vi "HMGET.vi"(8 "error in (no error)":errorcluster, 9 "fields":string[](array[string]), 10 "key":string, 11 "Redis Client in":refnum<class "Redis Client.lvclass">) -> (0 "error out":errorcluster, 1 "found?":bool, 2 "RESP3 Values out":variant[](array[variant]), 3 "Redis Client out":refnum<class "Redis Client.lvclass">)   [LabVIEW 2019, in "Redis Client for LabVIEW.lvlib" / "Redis Client.lvclass"]
uses:
  Redis Client.lvclass
  lib/RESP3-for-LabVIEW/RESP3/subVIs/RESP3 Make String Base.vi
  lib/RESP3-for-LabVIEW/RESP3/types/RESP3 data type attribute.vi
  lib/RESP3-for-LabVIEW/RESP3/RESP3.lvlib
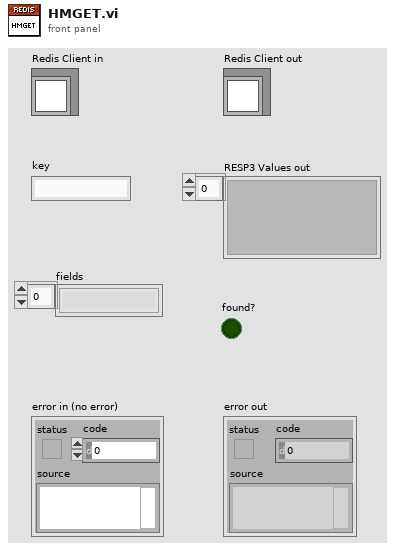
[diagram p1: front panel]
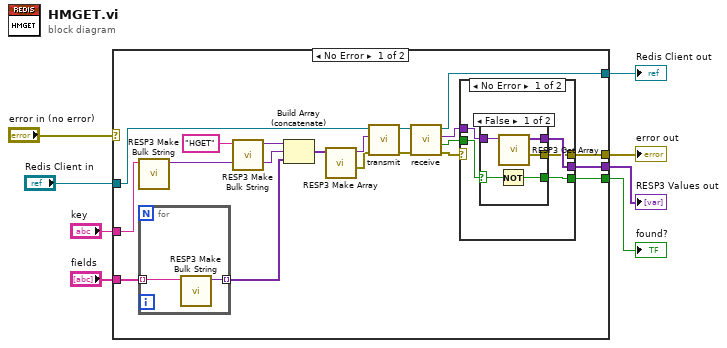
[diagram p0: block diagram]
diagram:
  n1 = case shown="No Error" "error in (no error)" {
    selector: "error in (no error)" -> [_ w42]
    tunnel: [w14 w42] -> w7
    tunnel: "Redis Client in" -> [w27 w41]
    tunnel: [w24 w41] -> w5
    tunnel: "key" -> [w21 _]
    tunnel: "fields" -> [w20 _]
    tunnel: [w13 _] -> w2
    tunnel: [w10 _] -> w1
    frame No Error {
      n2 = call "RESP3 Make Bulk String.vi"("String"=w21) -> ("RESP3 Value out"=w18:variant)  [unwired: 9 in, 1 out]
      n3 = for {
        tunnel: w20 -> [w29] mode=indexing
        tunnel: [w28] -> w17 mode=indexing
        n4 = call "RESP3 Make Bulk String.vi"("String"=w29) -> ("RESP3 Value out"=w28:variant)  [unwired: 9 in, 1 out]
      }
      n5 = call "RESP3 Make Bulk String.vi"("String"="HGET" ("string in")) -> ("RESP3 Value out"=w19:variant)  [unwired: 9 in, 1 out]
      n6 = Build Array (concatenate)(w19, w18, w17) -> (w26:variant[])
      n7 = call "RESP3 Make Array.vi"("RESP3 Values in"=w26) -> ("error out"=w15:errorcluster, "RESP3 Value out"=w16:variant)  [unwired: 9 in]
      n8 = call-dynamic "transmit.vi"("error in (no error)"=w15, "RESP3 Value"=w16, "Redis Client in"=w27) -> ("error out"=w23:errorcluster, "Redis Client out"=w25:refnum<class "Redis Client.lvclass">)  [unwired: 7 in]
      n9 = call-dynamic "receive.vi"("error in (no error)"=w23, "Redis Client in"=w25) -> ("error out"=w12:errorcluster, "timed out?"=w11:bool, "RESP3 Value"=w9:variant, "Redis Client out"=w24:refnum<class "Redis Client.lvclass">)  [unwired: 6 in]
      n10 = case shown="No Error" w12 {
        selector: w12 -> [_ w40]
        tunnel: [w31 w40] -> w14
        tunnel: [w34 _] -> w13
        tunnel: w11 -> [w33 _]
        tunnel: [w32 _] -> w10
        tunnel: w9 -> [w30 _]
        frame No Error {
          n11 = case shown="False" w33 {
            selector: w33 -> [w38 _]
            tunnel: w30 -> [w37 _]
            tunnel: [w39 _] -> w34
            tunnel: [w36 _] -> w32
            tunnel: [w35 _] -> w31
            frame False {
              n12 = Not(x=w38) -> (.not. x?=w39:bool)
              n13 = call "RESP3 Get Array.vi"("RESP3 Value in"=w37) -> ("error out"=w35:errorcluster, "RESP3 Values out"=w36:variant[])  [unwired: 7 in, 2 out]
            }
            frame True {
            }
          }
        }
        frame Error {
        }
      }
    }
    frame Error {
    }
  }
  "error out" <- w7
  "Redis Client out" <- w5
  "RESP3 Values out" <- w1
  "found?" <- w2
